vi "Spiral.vi"() -> ()   [LabVIEW 2016]
panel:
  in  "X Offset":dbl=257.0
  in  "Y Offset":dbl=77.0
  out "Waveform Graph":dbl[][](graph)=[[57.0, 59.5, 62.0, 64.5, 67.0, 69.5, 72.0, 74.5, 77.0, 79.5, 82.0, 84.5, 87.0, 89.5, 92.0, 94.5, 97.0, 97.0, 97.0, 97.0, 97.0, 97.0, 97.0, 97.0, 97.0, 97.0, 97.0, 97.0, 97.0, 97.0, 97.0, 97.0, 97.0, 97.0, 97.0, 94.5, 92.0, 89.5, 87.0, 84.5, 82.0, 79.5, 77.0, 74.5, 72.0, 69.5, 67.0, 64.5, 62.0, 59.5, 57.0, 57.0, 57.0, 57.0, 57.0, 57.0, 57.0, 57.0, 57.0, 57.0, 57.0, 57.0, 57.0, 57.0, 57.0, 57.0, 57.0, 59.5, 62.0, 64.5, 67.0, 69.5, 72.0, 74.5, 77.0, 79.5, 82.0, 84.5, 87.0, 89.5, 92.0, 94.5, 94.5, 94.5, 94.5, 94.5, 94.5, 94.5, 94.5, 94.5, 94.5, 94.5, 94.5, 94.5, 94.5, 94.5, 94.5, 94.5, 92.0, 89.5, 87.0, 84.5, 82.0, 79.5, 77.0, 74.5, 72.0, 69.5, 67.0, 64.5, 62.0, 59.5, 59.5, 59.5, 59.5, 59.5, 59.5, 59.5, 59.5, 59.5, 59.5, 59.5, 59.5, 59.5, 59.5, 59.5, 62.0, 64.5, 67.0, 69.5, 72.0, 74.5, 77.0, 79.5, 82.0, 84.5, 87.0, 89.5, 92.0, 92.0, 92.0, 92.0, 92.0, 92.0, 92.0, 92.0, 92.0, 92.0, 92.0, 92.0, 92.0, 92.0, 92.0, 89.5, 87.0, 84.5, 82.0, 79.5, 77.0, 74.5, 72.0, 69.5, 67.0, 64.5, 62.0, 62.0, 62.0, 62.0, 62.0, 62.0, 62.0, 62.0, 62.0, 62.0, 62.0, 62.0, 62.0, 64.5, 67.0, 69.5, 72.0, 74.5, 77.0, 79.5, 82.0, 84.5, 87.0, 89.5, 89.5, 89.5, 89.5, 89.5, 89.5, 89.5, 89.5, 89.5, 89.5, 89.5, 89.5, 89.5, 87.0, 84.5, 82.0, 79.5, 77.0, 74.5, 72.0, 69.5, 67.0, 64.5, 64.5, 64.5, 64.5, 64.5, 64.5, 64.5, 64.5, 64.5, 64.5, 64.5], [237.0, 237.0, 237.0, 237.0, 237.0, 237.0, 237.0, 237.0, 237.0, 237.0, 237.0, 237.0, 237.0, 237.0, 237.0, 237.0, 237.0, 237.0, 239.5, 242.0, 244.5, 247.0, 249.5, 252.0, 254.5, 257.0, 259.5, 262.0, 264.5, 267.0, 269.5, 272.0, 274.5, 277.0, 277.0, 277.0, 277.0, 277.0, 277.0, 277.0, 277.0, 277.0, 277.0, 277.0, 277.0, 277.0, 277.0, 277.0, 277.0, 277.0, 277.0, 277.0, 274.5, 272.0, 269.5, 267.0, 264.5, 262.0, 259.5, 257.0, 254.5, 252.0, 249.5, 247.0, 244.5, 242.0, 239.5, 239.5, 239.5, 239.5, 239.5, 239.5, 239.5, 239.5, 239.5, 239.5, 239.5, 239.5, 239.5, 239.5, 239.5, 239.5, 239.5, 242.0, 244.5, 247.0, 249.5, 252.0, 254.5, 257.0, 259.5, 262.0, 264.5, 267.0, 269.5, 272.0, 274.5, 274.5, 274.5, 274.5, 274.5, 274.5, 274.5, 274.5, 274.5, 274.5, 274.5, 274.5, 274.5, 274.5, 274.5, 274.5, 274.5, 272.0, 269.5, 267.0, 264.5, 262.0, 259.5, 257.0, 254.5, 252.0, 249.5, 247.0, 244.5, 242.0, 242.0, 242.0, 242.0, 242.0, 242.0, 242.0, 242.0, 242.0, 242.0, 242.0, 242.0, 242.0, 242.0, 242.0, 244.5, 247.0, 249.5, 252.0, 254.5, 257.0, 259.5, 262.0, 264.5, 267.0, 269.5, 272.0, 272.0, 272.0, 272.0, 272.0, 272.0, 272.0, 272.0, 272.0, 272.0, 272.0, 272.0, 272.0, 272.0, 272.0, 269.5, 267.0, 264.5, 262.0, 259.5, 257.0, 254.5, 252.0, 249.5, 247.0, 244.5, 244.5, 244.5, 244.5, 244.5, 244.5, 244.5, 244.5, 244.5, 244.5, 244.5, 244.5, 244.5, 247.0, 249.5, 252.0, 254.5, 257.0, 259.5, 262.0, 264.5, 267.0, 269.5, 269.5, 269.5, 269.5, 269.5, 269.5, 269.5, 269.5, 269.5, 269.5, 269.5, 269.5, 269.5, 267.0, 264.5, 262.0, 259.5, 257.0, 254.5, 252.0, 249.5, 247.0]]
  in  "Numeric":i32=4
  out "XY Graph":cluster{dbl[], dbl[]}(graph)={[57.0, 59.5, 62.0, 64.5, 67.0, 69.5, 72.0, 74.5, 77.0, 79.5, 82.0, 84.5, 87.0, 89.5, 92.0, 94.5, 97.0, 97.0, 97.0, 97.0, 97.0, 97.0, 97.0, 97.0, 97.0, 97.0, 97.0, 97.0, 97.0, 97.0, 97.0, 97.0, 97.0, 97.0, 97.0, 94.5, 92.0, 89.5, 87.0, 84.5, 82.0, 79.5, 77.0, 74.5, 72.0, 69.5, 67.0, 64.5, 62.0, 59.5, 57.0, 57.0, 57.0, 57.0, 57.0, 57.0, 57.0, 57.0, 57.0, 57.0, 57.0, 57.0, 57.0, 57.0, 57.0, 57.0, 57.0, 59.5, 62.0, 64.5, 67.0, 69.5, 72.0, 74.5, 77.0, 79.5, 82.0, 84.5, 87.0, 89.5, 92.0, 94.5, 94.5, 94.5, 94.5, 94.5, 94.5, 94.5, 94.5, 94.5, 94.5, 94.5, 94.5, 94.5, 94.5, 94.5, 94.5, 94.5, 92.0, 89.5, 87.0, 84.5, 82.0, 79.5, 77.0, 74.5, 72.0, 69.5, 67.0, 64.5, 62.0, 59.5, 59.5, 59.5, 59.5, 59.5, 59.5, 59.5, 59.5, 59.5, 59.5, 59.5, 59.5, 59.5, 59.5, 59.5, 62.0, 64.5, 67.0, 69.5, 72.0, 74.5, 77.0, 79.5, 82.0, 84.5, 87.0, 89.5, 92.0, 92.0, 92.0, 92.0, 92.0, 92.0, 92.0, 92.0, 92.0, 92.0, 92.0, 92.0, 92.0, 92.0, 92.0, 89.5, 87.0, 84.5, 82.0, 79.5, 77.0, 74.5, 72.0, 69.5, 67.0, 64.5, 62.0, 62.0, 62.0, 62.0, 62.0, 62.0, 62.0, 62.0, 62.0, 62.0, 62.0, 62.0, 62.0, 64.5, 67.0, 69.5, 72.0, 74.5, 77.0, 79.5, 82.0, 84.5, 87.0, 89.5, 89.5, 89.5, 89.5, 89.5, 89.5, 89.5, 89.5, 89.5, 89.5, 89.5, 89.5, 89.5, 87.0, 84.5, 82.0, 79.5, 77.0, 74.5, 72.0, 69.5, 67.0, 64.5, 64.5, 64.5, 64.5, 64.5, 64.5, 64.5, 64.5, 64.5, 64.5, 64.5], [237.0, 237.0, 237.0, 237.0, 237.0, 237.0, 237.0, 237.0, 237.0, 237.0, 237.0, 237.0, 237.0, 237.0, 237.0, 237.0, 237.0, 237.0, 239.5, 242.0, 244.5, 247.0, 249.5, 252.0, 254.5, 257.0, 259.5, 262.0, 264.5, 267.0, 269.5, 272.0, 274.5, 277.0, 277.0, 277.0, 277.0, 277.0, 277.0, 277.0, 277.0, 277.0, 277.0, 277.0, 277.0, 277.0, 277.0, 277.0, 277.0, 277.0, 277.0, 277.0, 274.5, 272.0, 269.5, 267.0, 264.5, 262.0, 259.5, 257.0, 254.5, 252.0, 249.5, 247.0, 244.5, 242.0, 239.5, 239.5, 239.5, 239.5, 239.5, 239.5, 239.5, 239.5, 239.5, 239.5, 239.5, 239.5, 239.5, 239.5, 239.5, 239.5, 239.5, 242.0, 244.5, 247.0, 249.5, 252.0, 254.5, 257.0, 259.5, 262.0, 264.5, 267.0, 269.5, 272.0, 274.5, 274.5, 274.5, 274.5, 274.5, 274.5, 274.5, 274.5, 274.5, 274.5, 274.5, 274.5, 274.5, 274.5, 274.5, 274.5, 274.5, 272.0, 269.5, 267.0, 264.5, 262.0, 259.5, 257.0, 254.5, 252.0, 249.5, 247.0, 244.5, 242.0, 242.0, 242.0, 242.0, 242.0, 242.0, 242.0, 242.0, 242.0, 242.0, 242.0, 242.0, 242.0, 242.0, 242.0, 244.5, 247.0, 249.5, 252.0, 254.5, 257.0, 259.5, 262.0, 264.5, 267.0, 269.5, 272.0, 272.0, 272.0, 272.0, 272.0, 272.0, 272.0, 272.0, 272.0, 272.0, 272.0, 272.0, 272.0, 272.0, 272.0, 269.5, 267.0, 264.5, 262.0, 259.5, 257.0, 254.5, 252.0, 249.5, 247.0, 244.5, 244.5, 244.5, 244.5, 244.5, 244.5, 244.5, 244.5, 244.5, 244.5, 244.5, 244.5, 244.5, 247.0, 249.5, 252.0, 254.5, 257.0, 259.5, 262.0, 264.5, 267.0, 269.5, 269.5, 269.5, 269.5, 269.5, 269.5, 269.5, 269.5, 269.5, 269.5, 269.5, 269.5, 269.5, 267.0, 264.5, 262.0, 259.5, 257.0, 254.5, 252.0, 249.5, 247.0]}
  in  "step size":dbl=2.5 format="%.4f"
  in  "Min":dbl=-20.0
  in  "Max":dbl=20.0
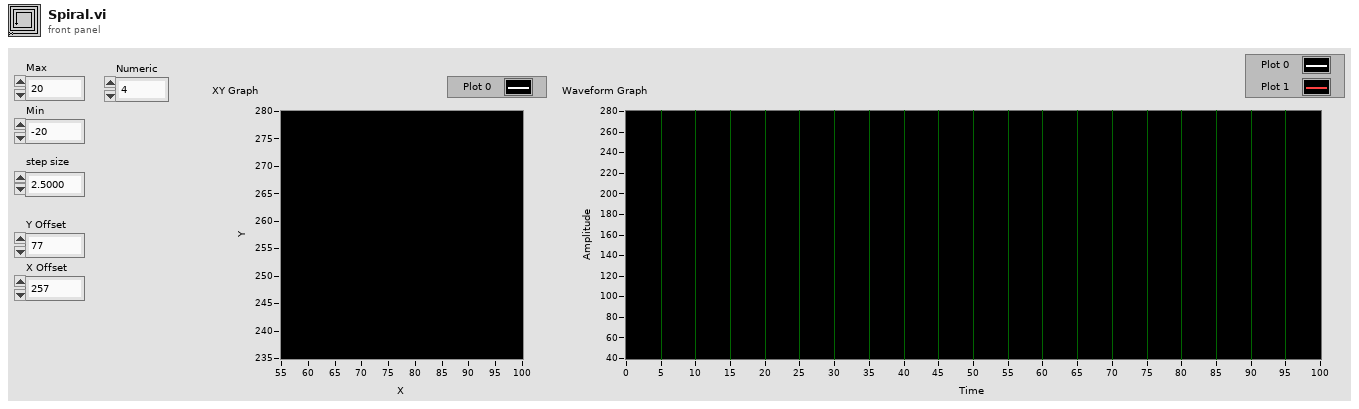
[diagram p1: front panel]
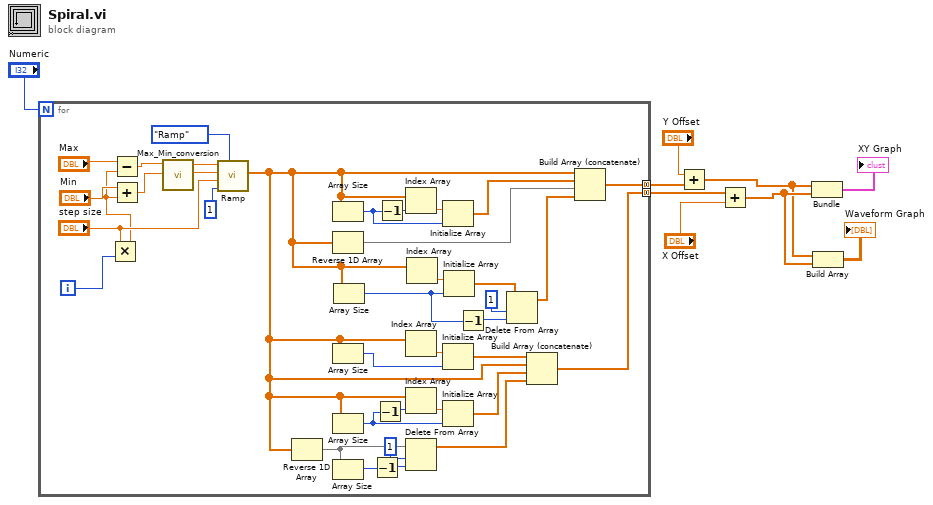
[diagram p0: block diagram]
diagram:
  n1 = for {
    N: "Numeric" -> [_]
    tunnel: [w42] -> w4 mode=concatenating
    tunnel: [w41] -> w1 mode=concatenating
    i -> [w18]
    n2 = Multiply(x="step size", y=w18) -> (x*y=w17:dbl)
    n3 = Subtract(x="Max", y=w17) -> (x-y=w15:dbl)
    n4 = Add(x="Min", y=w17) -> (x+y=w16:dbl)
    n5 = call <userlib>:"Max_Min_conversion.vi"("Min"=w16, "Max"=w15) -> ("offset"=w44:dbl, "Amplitude"=w45:dbl)  [unwired: 8 in]
    n6 = call <userlib>:"Ramp.vi"("function (ramp)"=enum16{"Ramp", "Triangle", "Sine"}."Ramp", "cycles (1,2,...)"=1, "step size"="step size", "offset"=w44, "amplitude"=w45) -> ("Waveform Graph"=w14:dbl[])  [unwired: 4 in, 2 out]
    n7 = Reverse 1D Array(array=w14) -> (reversed array=w26:dbl[])
    n8 = Array Size(array=w14) -> (size(s)=w11:i32)
    n9 = Reverse 1D Array(array=w14) -> (reversed array=w38:dbl[])
    n10 = Array Size(array=w14) -> (size(s)=w34:i32)
    n11 = Array Size(array=w14) -> (size(s)=w28:i32)
    n12 = Array Size(array=w26) -> (size(s)=w30:i32)
    n13 = Array Size(array=w14) -> (size(s)=w12:i32)
    n14 = Decrement(x=w30) -> (x-1=w31:i32)
    n15 = Decrement(x=w28) -> (x-1=w29:i32)
    n16 = Decrement(x=w11) -> (x-1=w24:i32)
    n17 = Index Array(array=w14, index=w24) -> (element=w40:dbl)
    n18 = Index Array(array=w14) -> (element=w37:dbl)  [unwired: 1 in]
    n19 = Index Array(array=w14, index=w29) -> (element=w35:dbl)
    n20 = Delete From Array(array=w26, length=1, index=w31) -> (array with subset deleted=w25:dbl[])  [unwired: 1 out]
    n21 = Index Array(array=w14) -> (element=w32:dbl)  [unwired: 1 in]
    n22 = Initialize Array(w40, w11) -> (w39:dbl[])
    n23 = Initialize Array(w37, w34) -> (w36:dbl[])
    n24 = Initialize Array(w35, w28) -> (w33:dbl[])
    n25 = Initialize Array(w32, w12) -> (w23:dbl[])
    n26 = Decrement(x=w12) -> (x-1=w13:i32)
    n27 = Delete From Array(array=w23, length=1, index=w13) -> (array with subset deleted=w10:dbl[])  [unwired: 1 out]
    n28 = Build Array (concatenate)(w36, w14, w33, w25) -> (w41:dbl[])
    n29 = Build Array (concatenate)(w14, w39, w38, w10) -> (w42:dbl[])
  }
  n30 = Add(x="Y Offset", y=w4) -> (x+y=w2:dbl[])
  n31 = Add(x=w1, y="X Offset") -> (x+y=w3:dbl[])
  n32 = Bundle(w2, w3) -> (→"XY Graph":cluster{dbl[], dbl[]})  [unwired: 1 in]
  n33 = Build Array(w2, w3) -> (→"Waveform Graph":dbl[][])
